vi "Processing Message Loop.vi"(8 "error in (no error)":errorcluster, 9 "Data Notifier":T2, 10 "Data Queue":T4, 11 "Message Queues":T5) -> (0 "error out":errorcluster)   [LabVIEW 2021, in "IMU Processing.lvlib"]
uses:
  IMU Processing.lvlib
  support/Message Queue/All Message Queues.ctl
  support/Message Queue/Message Cluster.ctl
  Acquisition/IMU Data Queue.ctl
  IMU TimeDataStruct.ctl
  <vilib>/silver_ctls/ArrayMatrixCluster/Real Matrix NI_Silver.ctl
  Acquisition/IMU Data Notifier.ctl
  Process state.ctl
  support/Message Queue/Enqueue Message (Single).vi
  ErrorModellingLibrary/VIs/Allan Variance Chart O.vi
  <vilib>/Utility/error.llb/Error Cluster From Error Code.vi
  <vilib>/ErrorRing/Error Ring.xnode
  support/Message Queue/IMU Message Queue.lvlib
  Logging/IMU Logging.lvlib
  ErrorModellingLibrary/ErrorModellingLibrary.lvlib
  <vilib>/gmath/NI_Gmath.lvlib
panel:
  in  "Calibrate":bool
  out "x-y":dbl[](array[numeric])
  out "x0, y0, z0":dbl[](array[numeric]) format="%.2f"
  in  "Acquire":i32=1000
  out "GyrZ":T1(array[cluster])
  out "GyrY":T1(array[cluster])
  out "GyrX":T1(array[cluster])
  out "AccZ":T1(array[cluster])
  out "AccY":T1(array[cluster])
  out "AccX":T1(array[cluster])
  out "n":i32[](array[numeric])
  in  "amount":u32=100
  out "Acquired":i32
  out "GyrY - Allan Variance":cluster{i32, "Numeric":dbl, "Numeric":dbl}[](graph)
  out "GyrX - Allan Variance":cluster{i32, "Numeric":dbl, "Numeric":dbl}[](graph)
  out "AccZ - Allan Variance":cluster{i32, "Numeric":dbl, "Numeric":dbl}[](graph)
  out "GyrZ - Allan Variance":cluster{i32, "Numeric":dbl, "Numeric":dbl}[](graph)
  out "AccY - Allan Variance":cluster{i32, "Numeric":dbl, "Numeric":dbl}[](graph)
  out "AccX - Allan Variance":cluster{i32, "Numeric":dbl, "Numeric":dbl}[](graph)
  out "Quaternion":dbl[](array[numeric])
  out "Rotation Matrix":T3
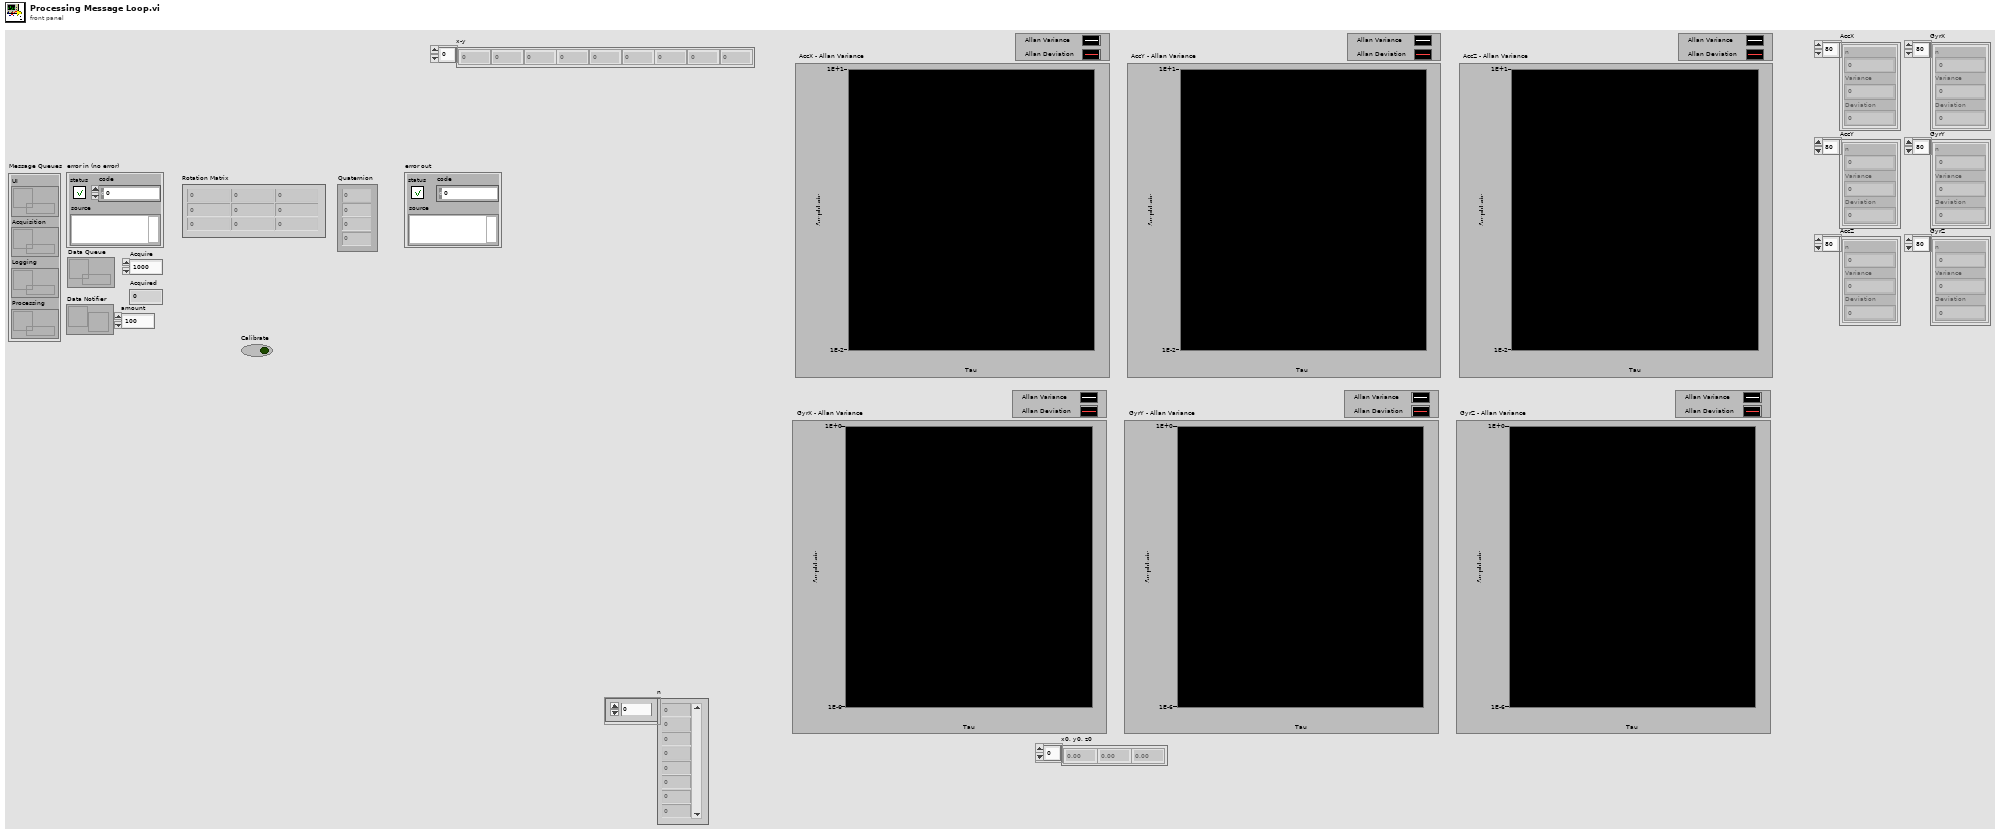
[diagram p1: front panel]
types:
  T1 = cluster{"n":i32, "Variance":dbl, "Deviation":dbl}[]
  T2 = typedef "IMU Data Notifier.ctl" = refnum<notifier>
  T3 = typedef "Real Matrix NI_Silver.ctl" = dbl[][]
  T4 = typedef "IMU Data Queue.ctl" = refnum<queue>
  T5 = typedef "IMU Message Queue.lvlib/All Message Queues.ctl" = cluster{"UI":refnum<queue>, "Acquisition":refnum<queue>, "Logging":refnum<queue>, "Processing":refnum<queue>}
  T6 = typedef "IMU Processing.lvlib/Process state.ctl" = enum16{"Idle", "Error Modelling", "Acquiring", "Processing"}
  T7 = typedef "IMU TimeDataStruct.ctl" = cluster{string, dbl[]}
  T8 = typedef "NI_Matrix.lvlib/RealMatrix.ctl" = dbl[][]
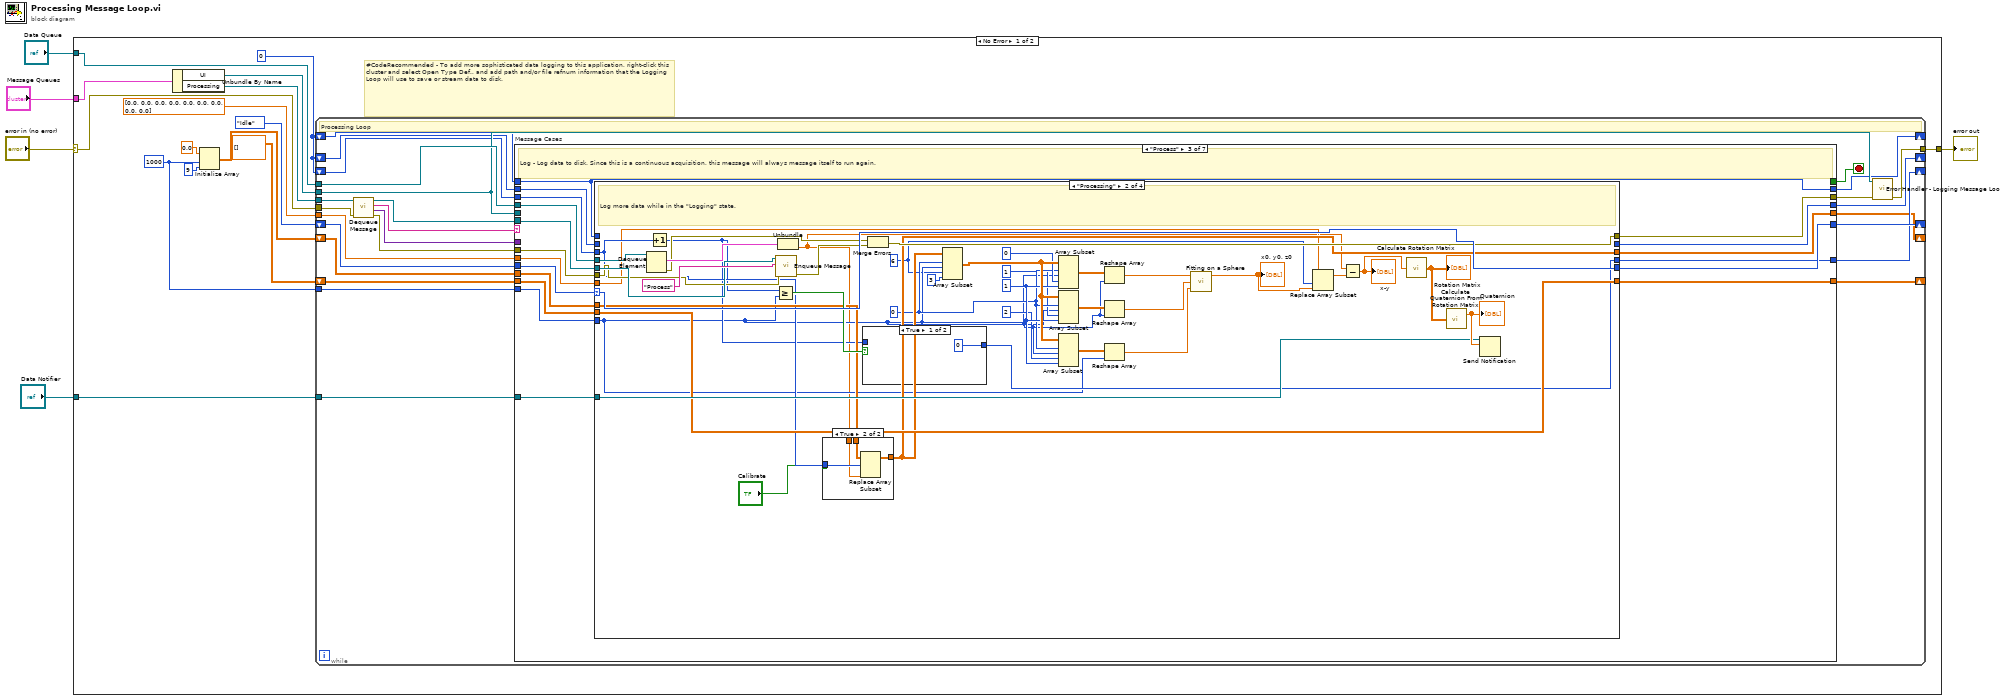
[diagram p0: block diagram]
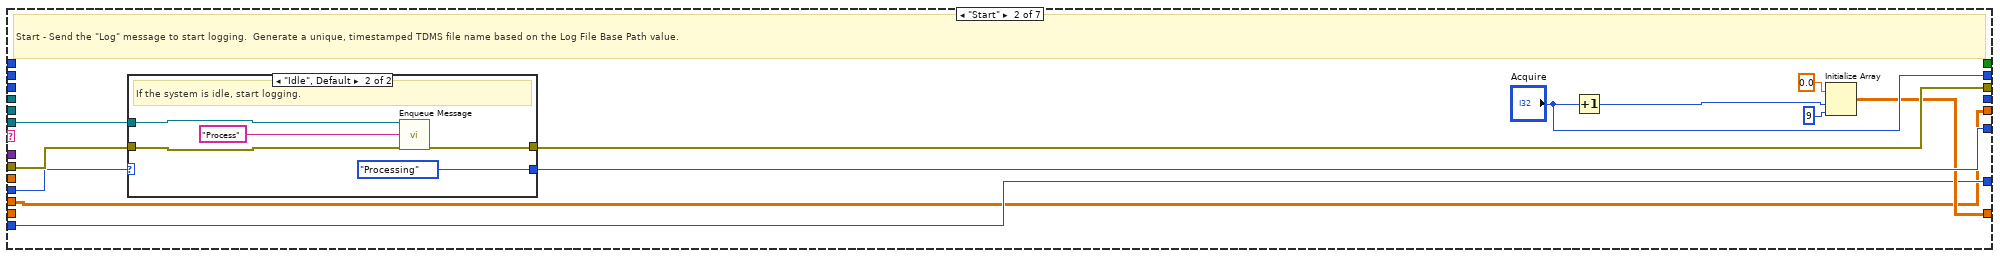
[diagram p3: hidden frame]
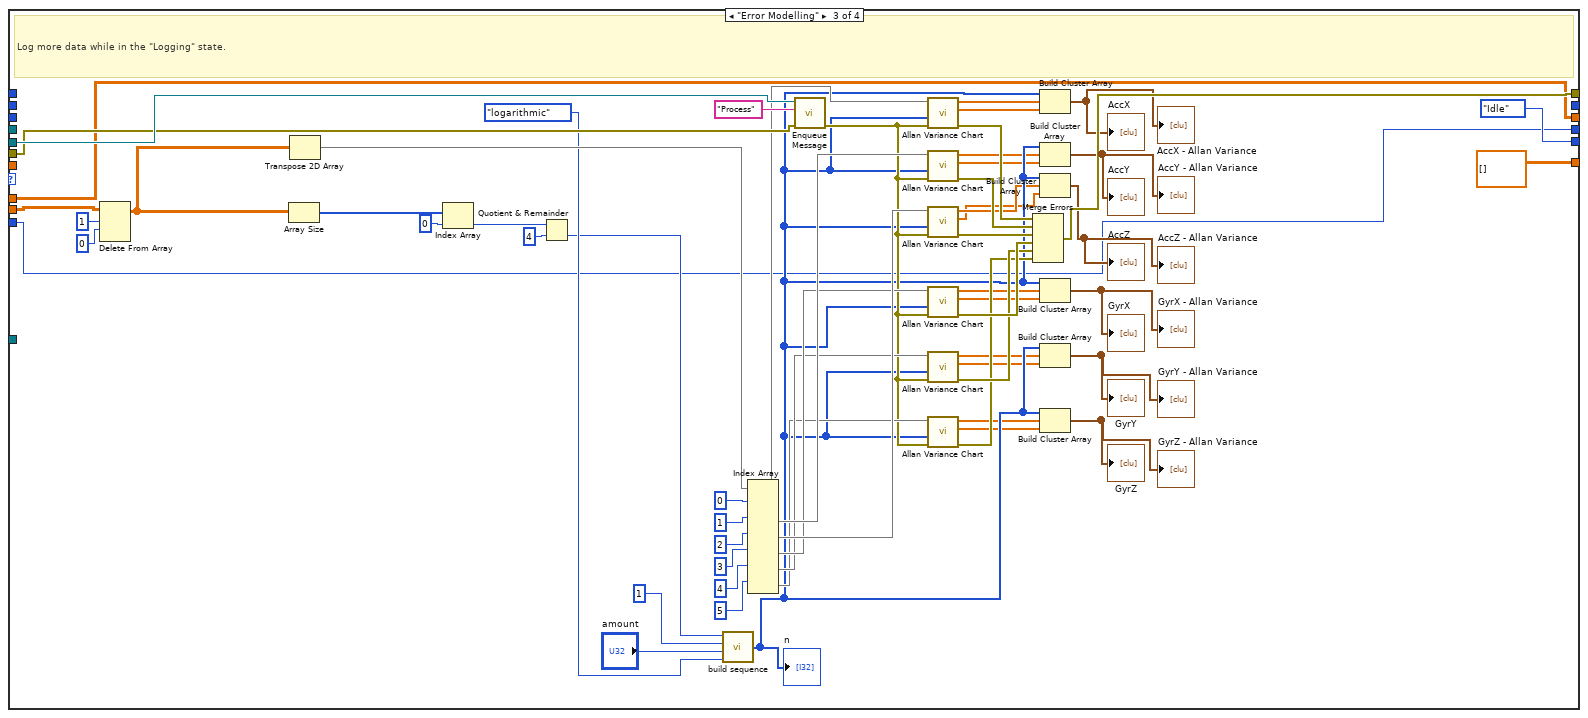
[diagram p8: hidden frame]
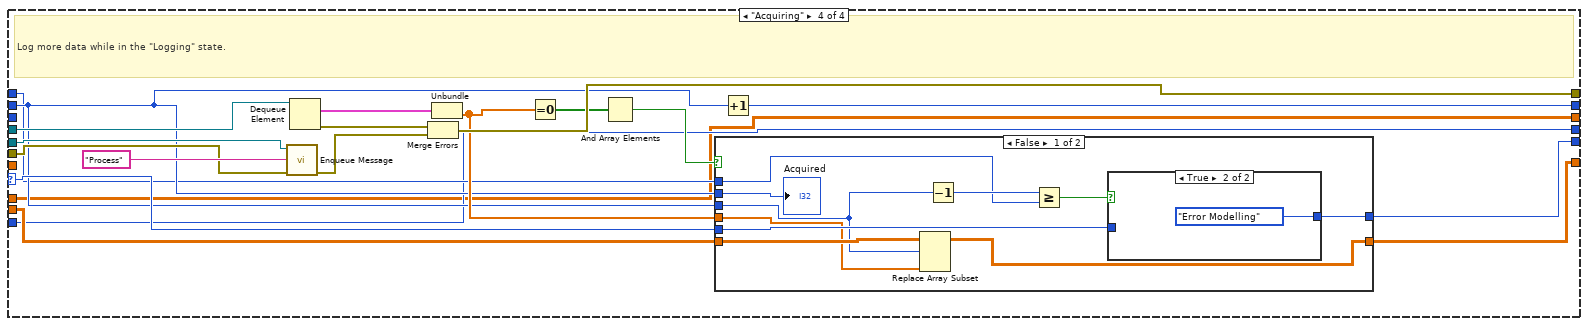
[diagram p9: hidden frame]
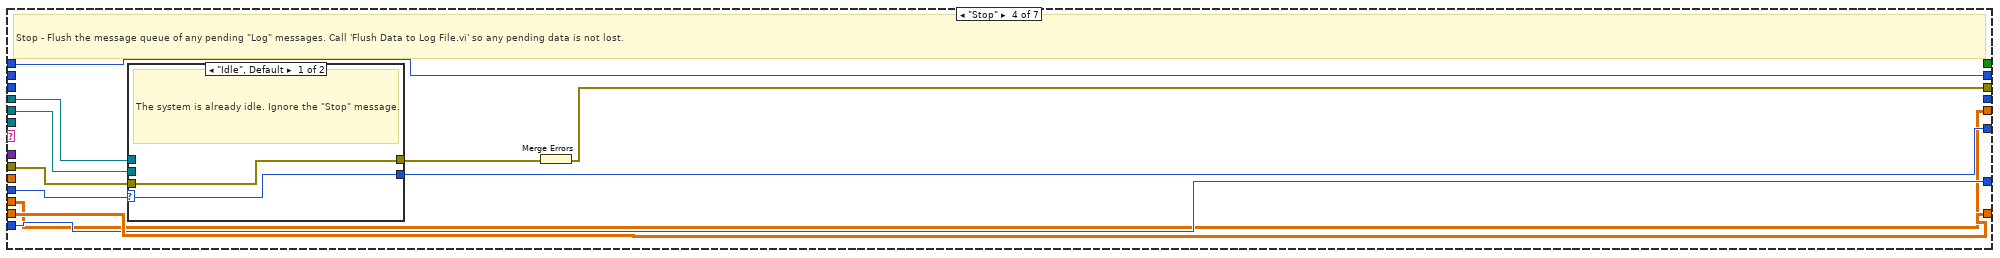
[diagram p12: hidden frame]
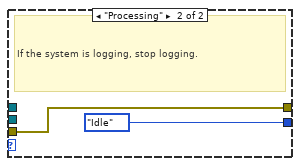
[diagram p13: hidden frame]
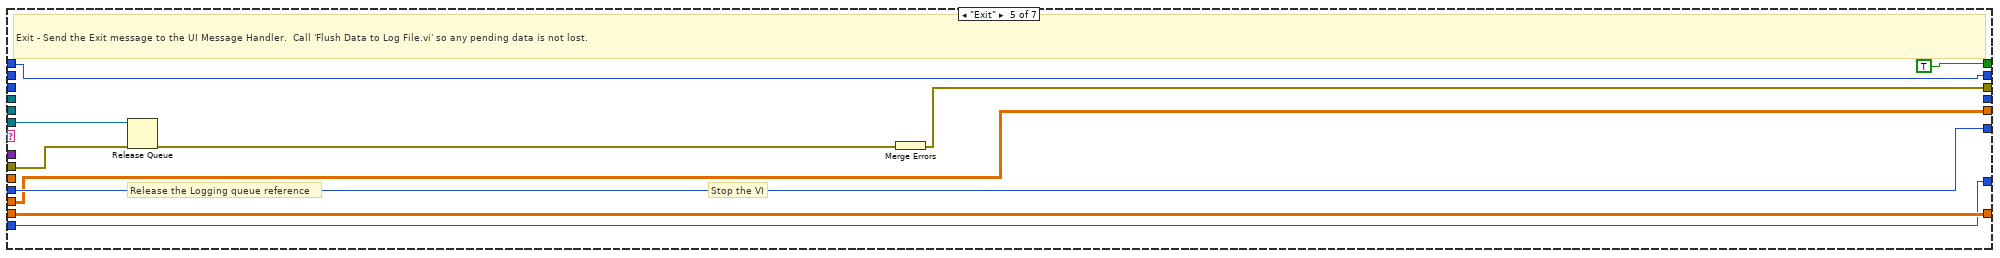
[diagram p14: hidden frame]
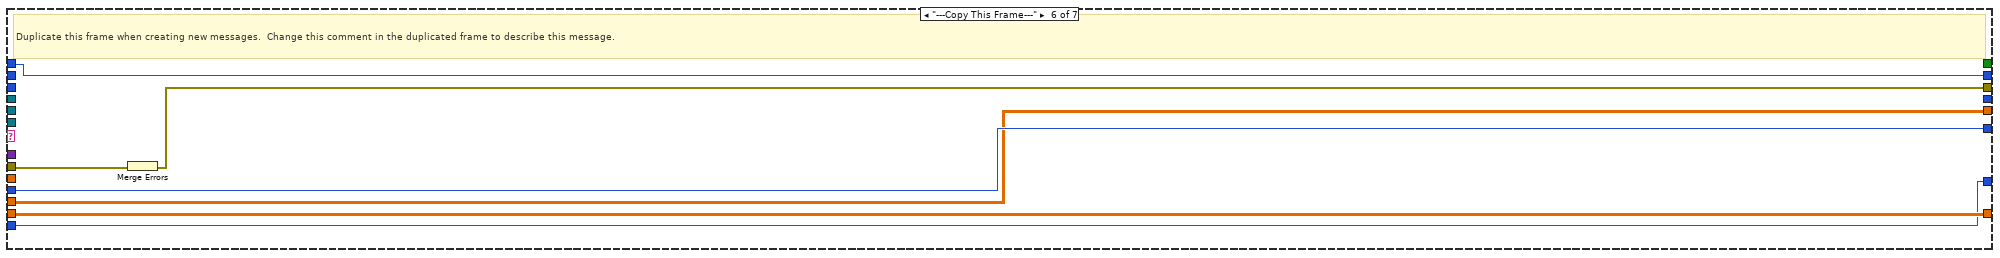
[diagram p15: hidden frame]
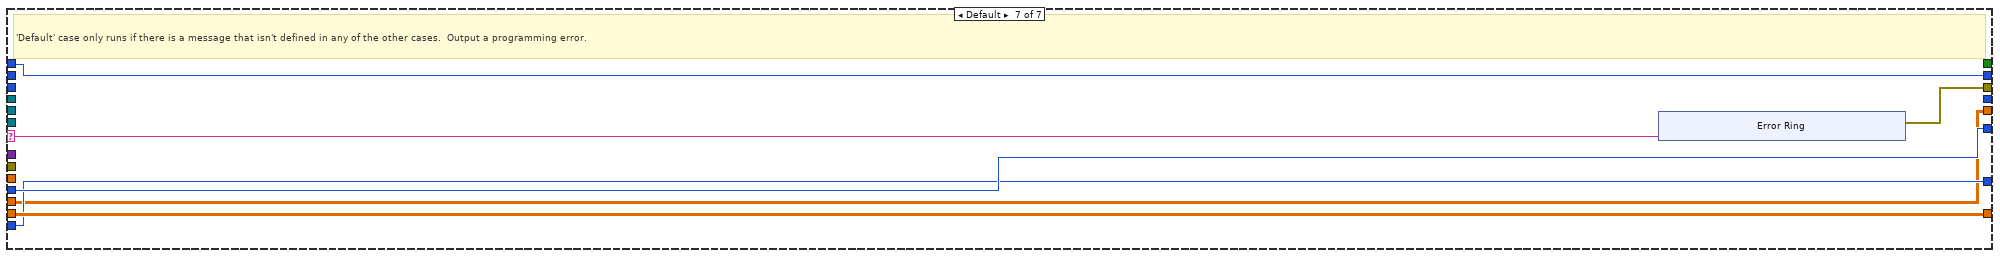
[diagram p16: hidden frame]
diagram:
  n1 = case shown="No Error" "error in (no error)" {
    selector: "error in (no error)" -> [w17 w281]
    tunnel: "Message Queues" -> [w20 _]
    tunnel: [w18 w281] -> w4
    tunnel: "Data Queue" -> [w16 _]
    tunnel: "Data Notifier" -> [w13 _]
    frame No Error {
      w8 = 1000 ("y")
      w12 = 0 ("Acquire")
      # "#CodeRecommended - To add more sophisticated data logging to this application, right-click this cluster and select Open Type Def., and add path and/or file refnum information that the Logging Loop will use to save or stream data to disk."
      n2 = Unbundle By Name(w20) -> ("UI"=w15:refnum<queue>, "Processing"=w19:refnum<queue>)
      n3 = Initialize Array(0.0 ("element"), w8, 9 ("dimension size")) -> (w9:dbl[][])
      n4 = while {
        tunnel: w19 -> [w40]
        tunnel: w15 -> [w34]
        tunnel: w16 -> [w39]
        shift-right: [w37] -> _
        shift-left: Process_state."Idle" ("Enum") -> [w38]
        tunnel: w17 -> [w45]
        tunnel: [w36] -> w18
        tunnel: w13 -> [w33]
        shift-right: [w32] -> _
        shift-left: dbl[][] [] -> [w31]
        shift-right: [w29] -> _
        shift-left: w12 -> [w30]
        shift-right: [w28] -> _
        shift-left: w12 -> [w27]
        shift-right: [w26] -> _
        shift-left: w12 -> [w25]
        tunnel: w8 -> [w24]
        shift-right: [w22] -> _
        shift-left: w9 -> [w23]
        tunnel: dbl[] [0.0, 0.0, 0.0, 0.0, 0.0, 0.0, 0.0, 0.0, 0.0] -> [w21]
        stop <- w46 stop-if-true
        # "Processing Loop"
        n5 = call "Dequeue Message.vi"("error in (no error)"=w45, "Message Queue"=w40) -> ("error out"=w44:errorcluster, "Message Data"=w42:variant, "Message"=w43:string, "dup Message Queue"=w41:refnum<queue>)  [unwired: 6 in]
        n6 = case "Message Cases" shown="\"Process\"" w43 {
          selector: w43 -> [_ _ _ _ _ _ w271]
          tunnel: w41 -> [_ w63 w88 _ w256 _ _]
          tunnel: w44 -> [w52 w62 w86 w242 w257 w266 _]
          tunnel: [w52 w64 w89 w245 w258 w265 w272] -> w35
          tunnel: [_ _ _ _ TRUE _ _] -> w46
          tunnel: w42 -> [_ _ _ _ _ _ _]
          tunnel: w34 -> [_ _ _ w239 _ _ _]
          tunnel: w39 -> [_ _ w87 w243 _ _ _]
          tunnel: w38 -> [w51 w61 w85 w241 w254 w264 w273]
          tunnel: [w51 w60 w84 w240 w254 w264 w273] -> w37
          tunnel: w33 -> [_ _ w83 _ _ _ _]
          tunnel: [w50 w56 w82 w238 w253 w263 w270] -> w32
          tunnel: w31 -> [w50 _ w81 w238 w253 w263 w270]
          tunnel: [w49 "Acquire" w78 w237 w252 w262 w269] -> w29
          tunnel: w30 -> [w49 _ w78 w237 w252 w262 w269]
          tunnel: [_ _ w80 _ _ _ _] -> w28
          tunnel: w27 -> [_ _ w79 _ _ _ _]
          tunnel: [w48 w54 w77 w236 w251 w261 w268] -> w26
          tunnel: w25 -> [_ _ w76 _ _ _ _]
          tunnel: w24 -> [w48 w54 w75 w236 w251 w261 w268]
          tunnel: w23 -> [w47 w53 w74 w235 w250 w260 w267]
          tunnel: [w47 w53 w73 w235 w250 w260 w267] -> w22
          tunnel: w21 -> [_ _ w72 _ _ _ _]
          frame "Initialize" {
            # "Initialize - gets called when first launched. Currently a no-op."
          }
          frame "Start" {
            # "Start - Send the \"Log\" message to start logging.  Generate a unique, timestamped TDMS file name based on the Log File Base Path value."
            n7 = case shown="\"Idle\", Default" w61 {
              selector: w61 -> [w66 _]
              tunnel: [w65 w67] -> w64
              tunnel: w63 -> [_ w69]
              tunnel: w62 -> [w65 w68]
              tunnel: [w66 Process_state."Processing" ("Enum")] -> w60
              frame "Processing" {
                # "The system is already logging. Ignore the \"Start\" message."
              }
              frame "Idle", Default {
                # "If the system is idle, start logging."
                n8 = call-poly "Enqueue Message.vi"("error in (no error)"=w68, "Message"="Process", "Message Queue"=w69) -> ("error out"=w67:errorcluster)  [unwired: 7 in, 1 out]
              }
            }
            n9 = Increment(x="Acquire") -> (x+1=w55:i32)
            n10 = Initialize Array(0.0 ("element"), w55, 9 ("dimension size")) -> (w56:dbl[][])
          }
          frame "Process" {
            # "Log - Log data to disk. Since this is a continuous acquisition, this message will always message itself to run again."
            n11 = case shown="\"Processing\"" w85 {
              selector: w85 -> [w94 w134 _ w212]
              tunnel: [w93 w127 w186 w214] -> w89
              tunnel: w88 -> [_ w132 w199 w219]
              tunnel: w87 -> [_ w130 _ w217]
              tunnel: w86 -> [w93 w128 w194 w215]
              tunnel: [w94 w134 Process_state."Idle" ("Enum") w211] -> w84
              tunnel: w83 -> [_ w123 _ _]
              tunnel: [w92 w122 dbl[][] [] w209] -> w82
              tunnel: w81 -> [w92 w122 w198 w210]
              tunnel: [_ _ _ w205] -> w80
              tunnel: w79 -> [_ _ _ w204]
              tunnel: w78 -> [_ _ _ w203]
              tunnel: [w91 w120 w143 w202] -> w77
              tunnel: w76 -> [_ w118 _ _]
              tunnel: w75 -> [w91 w103 w143 w202]
              tunnel: w74 -> [w90 w119 w142 w201]
              tunnel: [w90 w116 w142 w201] -> w73
              tunnel: w72 -> [_ w99 _ _]
              frame "Idle" {
                # "Ignore \"Log\" messages when the logging is idle."
              }
              frame "Processing" {
                w101 = 6 ("index")
                w110 = 1 ("length")
                w109 = 0 ("index")
                # "Log more data while in the \"Logging\" state."
                n12 = Dequeue Element(queue=w130) -> (element=w131:T7, error out=w126:errorcluster)  [unwired: 2 in, 2 out]
                n13 = Increment(x=w118) -> (x+1=w117:i32)
                n14 = Greater Or Equal?(x=w117, y=w103) -> (x >= y?=w121:bool)
                n15 = call-poly "Enqueue Message.vi"("error in (no error)"=w128, "Message"="Process", "Message Queue"=w132) -> ("error out"=w129:errorcluster)  [unwired: 7 in, 1 out]
                n16 = Unbundle(w131) -> (w98:dbl[])  [unwired: 1 out]
                n17 = case shown="True" "Calibrate" {
                  tunnel: w119 -> [w135 w139]
                  tunnel: w118 -> [_ w138]
                  tunnel: [w135 w137] -> w116
                  tunnel: w98 -> [_ w136]
                  frame False {
                  }
                  frame True {
                    n18 = Replace Array Subset(array=w139, new element=w136, index (row)=w138) -> (w137:dbl[][])  [unwired: 1 in]
                  }
                }
                n19 = case shown="True" w121 {
                  tunnel: w117 -> [_ w141]
                  tunnel: [0 w141] -> w120
                  frame True {
                  }
                  frame False {
                  }
                }
                n20 = Merge Errors(w126, w129) -> (w127:errorcluster)
                n21 = Array Subset(array=w116, index (row)=w109, length (row)=w103, index (col)=w101, length (col)=3 ("length")) -> (w112:dbl[][])
                n22 = Array Subset(array=w112, index (row)=w109, length (row)=w103, index (col)=0 ("index"), length (col)=w110) -> (w115:dbl[][])
                n23 = Array Subset(array=w112, index (row)=w109, length (row)=w103, index (col)=1 ("index"), length (col)=w110) -> (w114:dbl[][])
                n24 = Array Subset(array=w112, index (row)=w109, length (row)=w103, index (col)=2 ("index"), length (col)=w110) -> (w113:dbl[][])
                n25 = Reshape Array(w115, w103) -> (w106:dbl[])
                n26 = Reshape Array(w114, w103) -> (w105:dbl[])
                n27 = Reshape Array(w113, w103) -> (w104:dbl[])
                n28 = call <vilib>:"Fitting on a Sphere.vi"("Z"=w104, "Y"=w105, "X"=w106) -> ("x0, y0, z0"=w102:dbl[])  [unwired: 2 out]
                "x0, y0, z0" <- w102
                n29 = Replace Array Subset(array=w99, new element=w102, index=w101) -> (w97:dbl[])
                n30 = Subtract(x=w98, y=w97) -> (x-y=w96:dbl[])
                "x-y" <- w96
                n31 = call "Calculate Rotation Matrix.vi"("data AGM - XYZ"=w96) -> ("Rotation Matrix"=w125:T8)
                "Rotation Matrix" <- w125
                n32 = call "Calculate Quaternion From Rotation Matrix.vi"("Rotation Matrix"=w125) -> ("appended array"=w124:dbl[])  [unwired: 1 out]
                "Quaternion" <- w124
                n33 = Send Notification(notification=w124, notifier=w123) -> ()  [unwired: 1 in, 2 out]
              }
              frame "Error Modelling" {
                # "Log more data while in the \"Logging\" state."
                n34 = Delete From Array(array=w198, length=1, index (row)=0) -> (array with subset deleted=w171:dbl[][])  [unwired: 1 in, 1 out]
                n35 = Array Size(array=w171) -> (size(s)=w170:i32[])
                n36 = Transpose 2D Array(2D array=w171) -> (transposed array=w197:dbl[][])
                n37 = Index Array(array=w170, index=0) -> (element=w168:i32)
                n38 = Quotient & Remainder(x=w168, y=4) -> (floor(x/y)=w163:i32)  [unwired: 1 out]
                n39 = call "build sequence.vi"("Enum"=enum16{"logarithmic", "linear"}."logarithmic", "amount"="amount", "min"=u32 1, "max"=w163) -> ("Array - Numeric"=w159:i32[])
                "n" <- w159
                n40 = Index Array(array=w197, index (row) #1=0 ("index (row)"), index (row) #2=1 ("index (row)"), index (row) #3=2 ("index (row)"), index (row) #4=3 ("index (row)"), index (row) #5=4 ("index (row)"), index (row) #6=5 ("index (row)")) -> (element #1=w185:dbl[], element #2=w183:dbl[], element #3=w182:dbl[], element #4=w181:dbl[], element #5=w180:dbl[], element #6=w179:dbl[])  [unwired: 6 in]
                n41 = call-poly "Enqueue Message.vi"("error in (no error)"=w194, "Message"="Process", "Message Queue"=w199) -> ("error out"=w178:errorcluster)  [unwired: 7 in, 1 out]
                n42 = call-poly "Allan Variance Chart.vi"("error in (no error)"=w178, "nArray"=w159, "inputdata"=w185) -> ("error out"=w184:errorcluster, "Allan Deviation"=w161:dbl[], "Allan Variance"=w162:dbl[])  [unwired: 6 in]
                n43 = call-poly "Allan Variance Chart.vi"("error in (no error)"=w178, "nArray"=w159, "inputdata"=w183) -> ("error out"=w177:errorcluster, "Allan Deviation"=w157:dbl[], "Allan Variance"=w158:dbl[])  [unwired: 6 in]
                n44 = call-poly "Allan Variance Chart.vi"("error in (no error)"=w178, "nArray"=w159, "inputdata"=w182) -> ("error out"=w176:errorcluster, "Allan Deviation"=w155:dbl[], "Allan Variance"=w156:dbl[])  [unwired: 6 in]
                n45 = call-poly "Allan Variance Chart.vi"("error in (no error)"=w178, "nArray"=w159, "inputdata"=w181) -> ("error out"=w175:errorcluster, "Allan Deviation"=w153:dbl[], "Allan Variance"=w154:dbl[])  [unwired: 6 in]
                n46 = call-poly "Allan Variance Chart.vi"("error in (no error)"=w178, "nArray"=w159, "inputdata"=w180) -> ("error out"=w174:errorcluster, "Allan Deviation"=w151:dbl[], "Allan Variance"=w152:dbl[])  [unwired: 6 in]
                n47 = call-poly "Allan Variance Chart.vi"("error in (no error)"=w178, "nArray"=w159, "inputdata"=w179) -> ("error out"=w173:errorcluster, "Allan Deviation"=w149:dbl[], "Allan Variance"=w150:dbl[])  [unwired: 6 in]
                n48 = Merge Errors(w184, w177, w176, w175, w174, w173) -> (w186:errorcluster)
                n49 = Build Cluster Array(w159, w162, w161) -> (→"AccX - Allan Variance" →"AccX":cluster{i32, "Numeric":dbl, "Numeric":dbl}[])
                n50 = Build Cluster Array(w159, w158, w157) -> (→"AccY - Allan Variance" →"AccY":cluster{i32, "Numeric":dbl, "Numeric":dbl}[])
                n51 = Build Cluster Array(w159, w156, w155) -> (→"AccZ - Allan Variance" →"AccZ":cluster{i32, "Numeric":dbl, "Numeric":dbl}[])
                n52 = Build Cluster Array(w159, w154, w153) -> (→"GyrX - Allan Variance" →"GyrX":cluster{i32, "Numeric":dbl, "Numeric":dbl}[])
                n53 = Build Cluster Array(w159, w152, w151) -> (→"GyrY - Allan Variance" →"GyrY":cluster{i32, "Numeric":dbl, "Numeric":dbl}[])
                n54 = Build Cluster Array(w159, w150, w149) -> (→"GyrZ - Allan Variance" →"GyrZ":cluster{i32, "Numeric":dbl, "Numeric":dbl}[])
              }
              frame "Acquiring" {
                # "Log more data while in the \"Logging\" state."
                n55 = call-poly "Enqueue Message.vi"("error in (no error)"=w215, "Message"="Process", "Message Queue"=w219) -> ("error out"=w216:errorcluster)  [unwired: 7 in, 1 out]
                n56 = Dequeue Element(queue=w217) -> (element=w218:T7, error out=w213:errorcluster)  [unwired: 2 in, 2 out]
                n57 = Merge Errors(w213, w216) -> (w214:errorcluster)
                n58 = Unbundle(w218) -> (w206:dbl[])  [unwired: 1 out]
                n59 = Equal To 0?(x=w206) -> (x = 0?=w208:bool[])
                n60 = And Array Elements(Boolean array=w208) -> (logical AND=w207:bool)
                n61 = case shown="False" w207 {
                  tunnel: w212 -> [w230 w233]
                  tunnel: [w229 w233] -> w211
                  tunnel: w210 -> [w228 w234]
                  tunnel: [w227 w234] -> w209
                  tunnel: w206 -> [w224 _]
                  tunnel: w204 -> [w225 _]
                  tunnel: w204 -> [w223 _]
                  tunnel: w203 -> [w221 _]
                  frame False {
                    n62 = Replace Array Subset(array=w228, new element=w224, index (row)=w225) -> (w227:dbl[][])  [unwired: 1 in]
                    n63 = Decrement(x=w225) -> (x-1=w222:i32)
                    n64 = Greater Or Equal?(x=w222, y=w221) -> (x >= y?=w226:bool)
                    n65 = case shown="True" w226 {
                      tunnel: w230 -> [w231 _]
                      tunnel: [w231 Process_state."Error Modelling" ("Enum")] -> w229
                      frame False {
                      }
                      frame True {
                      }
                    }
                    "Acquired" <- w223
                  }
                  frame True {
                  }
                }
                n66 = Increment(x=w204) -> (x+1=w205:i32)
              }
            }
          }
          frame "Stop" {
            # "Stop - Flush the message queue of any pending \"Log\" messages. Call 'Flush Data to Log File.vi' so any pending data is not lost."
            n67 = case shown="\"Idle\", Default" w241 {
              selector: w241 -> [w246 _]
              tunnel: [w247 w248] -> w244
              tunnel: w243 -> [_ _]
              tunnel: w242 -> [w247 w248]
              tunnel: [w246 Process_state."Idle" ("Enum")] -> w240
              tunnel: w239 -> [_ _]
              frame "Idle", Default {
                # "The system is already idle. Ignore the \"Stop\" message."
              }
              frame "Processing" {
                # "If the system is logging, stop logging."
              }
            }
            n68 = Merge Errors(w244) -> (w245:errorcluster)
          }
          frame "Exit" {
            # "Release the Logging queue reference"
            # "Stop the VI"
            # "Exit - Send the Exit message to the UI Message Handler.  Call 'Flush Data to Log File.vi' so any pending data is not lost."
            n69 = Release Queue(queue=w256, error in (no error)=w257) -> (error out=w255:errorcluster)  [unwired: 1 in, 2 out]
            n70 = Merge Errors(w255) -> (w258:errorcluster)
          }
          frame "---Copy This Frame---" {
            # "Duplicate this frame when creating new messages.  Change this comment in the duplicated frame to describe this message."
            n71 = Merge Errors(w266) -> (w265:errorcluster)
          }
          frame Default {
            # "'Default' case only runs if there is a message that isn't defined in any of the other cases.  Output a programming error."
            n72 = xnode "Error Ring"("parameter 0"=w271) -> ("error out"=w272:errorcluster)
          }
        }
        n73 = call "Error Handler - Logging Message Loop.vi"("error in (no error)"=w35, "Message Queue"=w34) -> ("dup error in"=w36:errorcluster)  [unwired: 8 in, 1 out]
      }
    }
    frame Error {
    }
  }
  "error out" <- w4
